vi "writeToXML.vi"(8 "error in (no error)":errorcluster, 10 "Class Label":string="SunMoonStatus", 11 "SunMoonStatus in":refnum<class "SunMoonStatus.lvclass">) -> (0 "error out":errorcluster, 2 "XML out":string="<SunMoonStatus>\n  <distance_deg>0</distance_deg>\n  <proximityFlag>false</proximityFlag>\n</SunMoonStatus>", 3 "SunMoonStatus out":refnum<class "SunMoonStatus.lvclass">)   [LabVIEW 2014, in "TCSDataDefinitions.lvlib" / "TCSPublicStatus.lvlib" / "Limits.lvlib" / "SunMoonStatus.lvclass"]
uses:
  SunMoonStatus.lvclass
  <userlib>/Common/UnitsAndXML/FlattenItemWithUnitToXML/FlattenPlaneAngleToXML/PlaneAngleUnit.ctl
  SunMoonStatus.lvclass/SunMoonStatus.ctl
  <userlib>/Common/UnitsAndXML/UnitsAndXML.lvlib
  <userlib>/Common/XML/XMLGenerator/XMLGenerator.lvclass
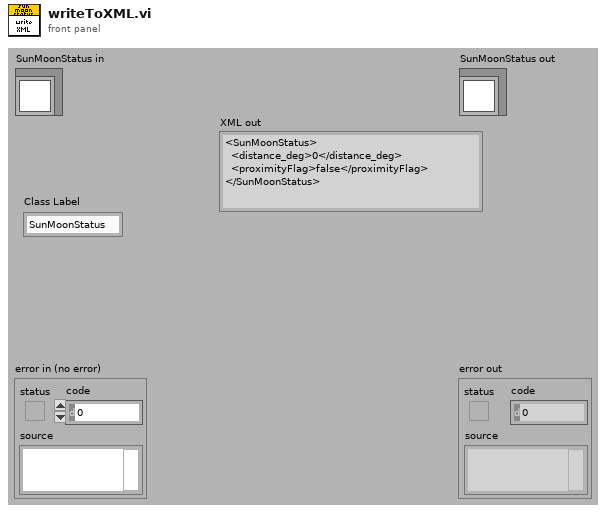
[diagram p1: front panel]
types:
  T1 = typedef "UnitsAndXML.lvlib/PlaneAngleUnit.ctl" = enum16{"rad", "deg", "'", "\""}
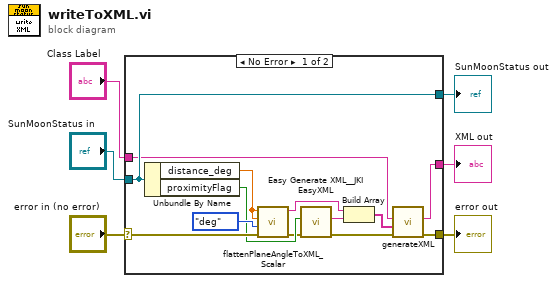
[diagram p0: block diagram]
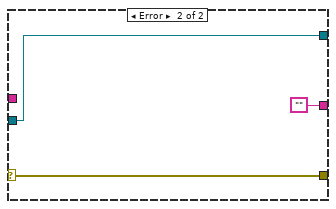
[diagram p2: hidden frame]
diagram:
  n1 = case shown="No Error" "error in (no error)" {
    selector: "error in (no error)" -> [w13 w22]
    tunnel: [w12 w22] -> w5
    tunnel: [w19 w21] -> w3
    tunnel: "SunMoonStatus in" -> [w19 w21]
    tunnel: "Class Label" -> [w14 _]
    tunnel: [w11 ""] -> w1
    frame No Error {
      n2 = Unbundle By Name(w19) -> ("distance_deg"=w18:dbl[unit], "proximityFlag"=w10:bool)
      n3 = call <userlib>:"flattenPlaneAngleToXML_Scalar.vi"("error in (no error)"=w13, "planeAngleUnitInXML"=PlaneAngleUnit."deg", "planeAngleAgain"=w18, "planeAngle"=w18) -> ("error out"=w9:errorcluster, "xmlString"=w16:string)  [unwired: 6 in]
      n4 = call <vilib>:"Easy Generate XML__JKI EasyXML.vi"("error in (no error)"=w9, "LabVIEW Data"=w10) -> ("error out"=w8:errorcluster, "XML String"=w7:string)  [unwired: 8 in]
      n5 = Build Array(w16, w7) -> (w15:string[])
      n6 = call <userlib>:"generateXML.vi"("error in"=w8, "childrenXML"=w15, "elementName"=w14) -> ("error out"=w12:errorcluster, "XML out"=w11:string)  [unwired: 6 in, 1 out]
    }
    frame Error {
    }
  }
  "error out" <- w5
  "SunMoonStatus out" <- w3
  "XML out" <- w1
